vi "loadEntityTransaction.vi"() -> ()   [LabVIEW 2012]
uses:
  <vilib>/addons/database/Connection.llb/DB Tools Open Connec (Path).vi
  <vilib>/addons/database/Connection.llb/Conn Execute.vi
  <vilib>/addons/database/Recordset.llb/Rec Fetch Recordset Data (R).vi
  <vilib>/addons/database/Recordset.llb/Rec Destroy - Connection.vi
  <vilib>/addons/database/_DB Variant To Data/Database Variant To Data.xnode
  <vilib>/addons/database/NI_Database_API.lvlib
panel:
  out "recordset data":variant[][](array[variant])
  out "error out 3":errorcluster
  out "data 2":string
  out "error out 2":errorcluster
  in  "Cluster":T1
  out "concatenated string":string
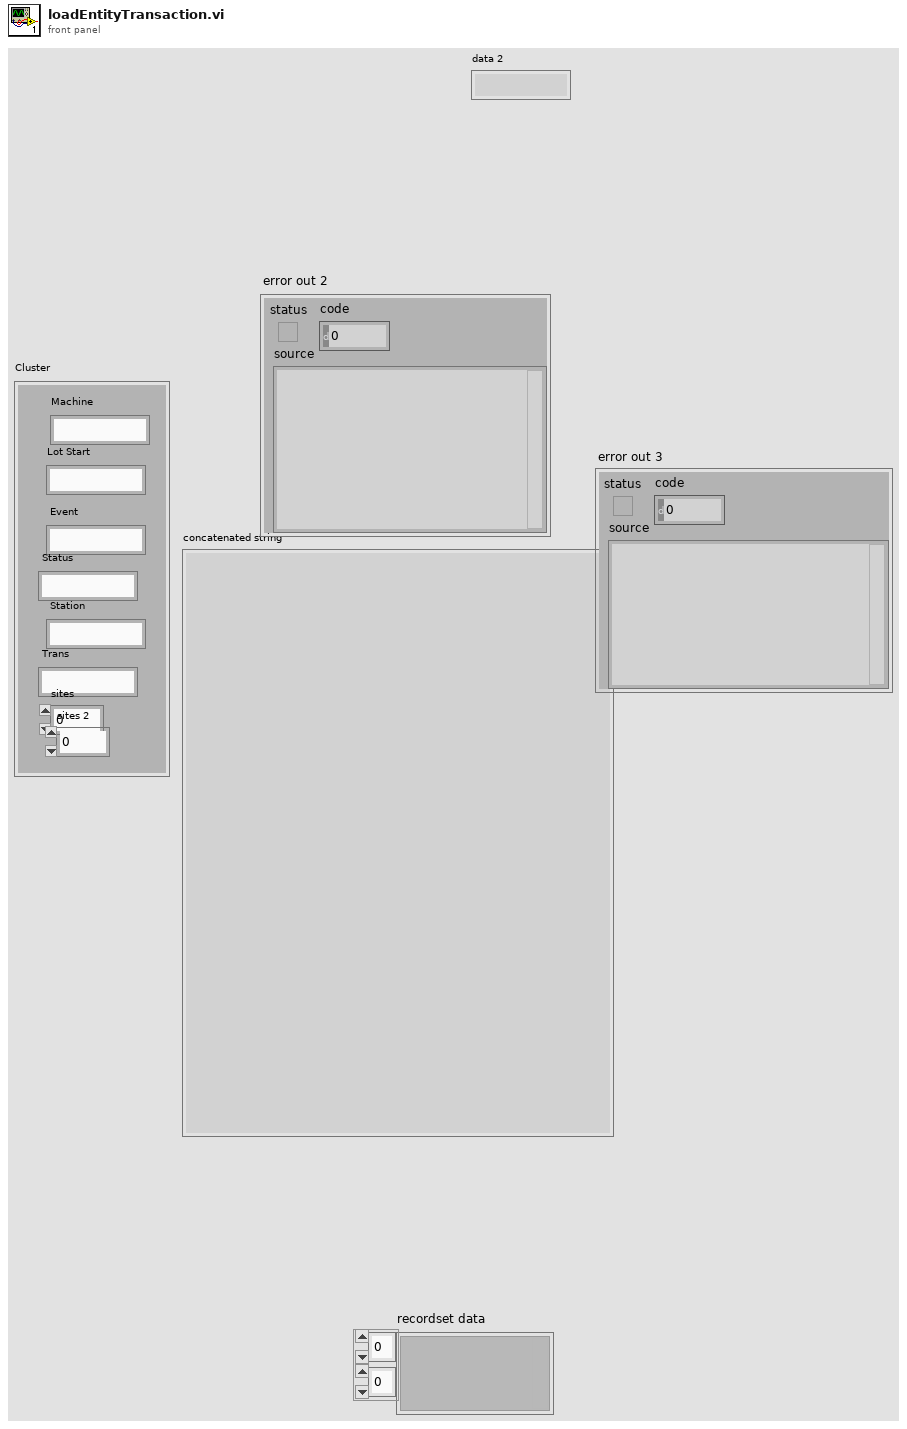
[diagram p1: front panel]
types:
  T1 = cluster{"Machine":string, "Lot Start":string, " Event":string, " Status":string, " Station":string, " Trans":string, "sites":dbl, "sites 2":dbl}
  T2 = typedef "NI_Database_API.lvlib/Conn ObjectReference.ctl" = refnum<k1>
  T3 = typedef "NI_Database_API.lvlib/Rec ObjectReference.ctl" = refnum<k1>
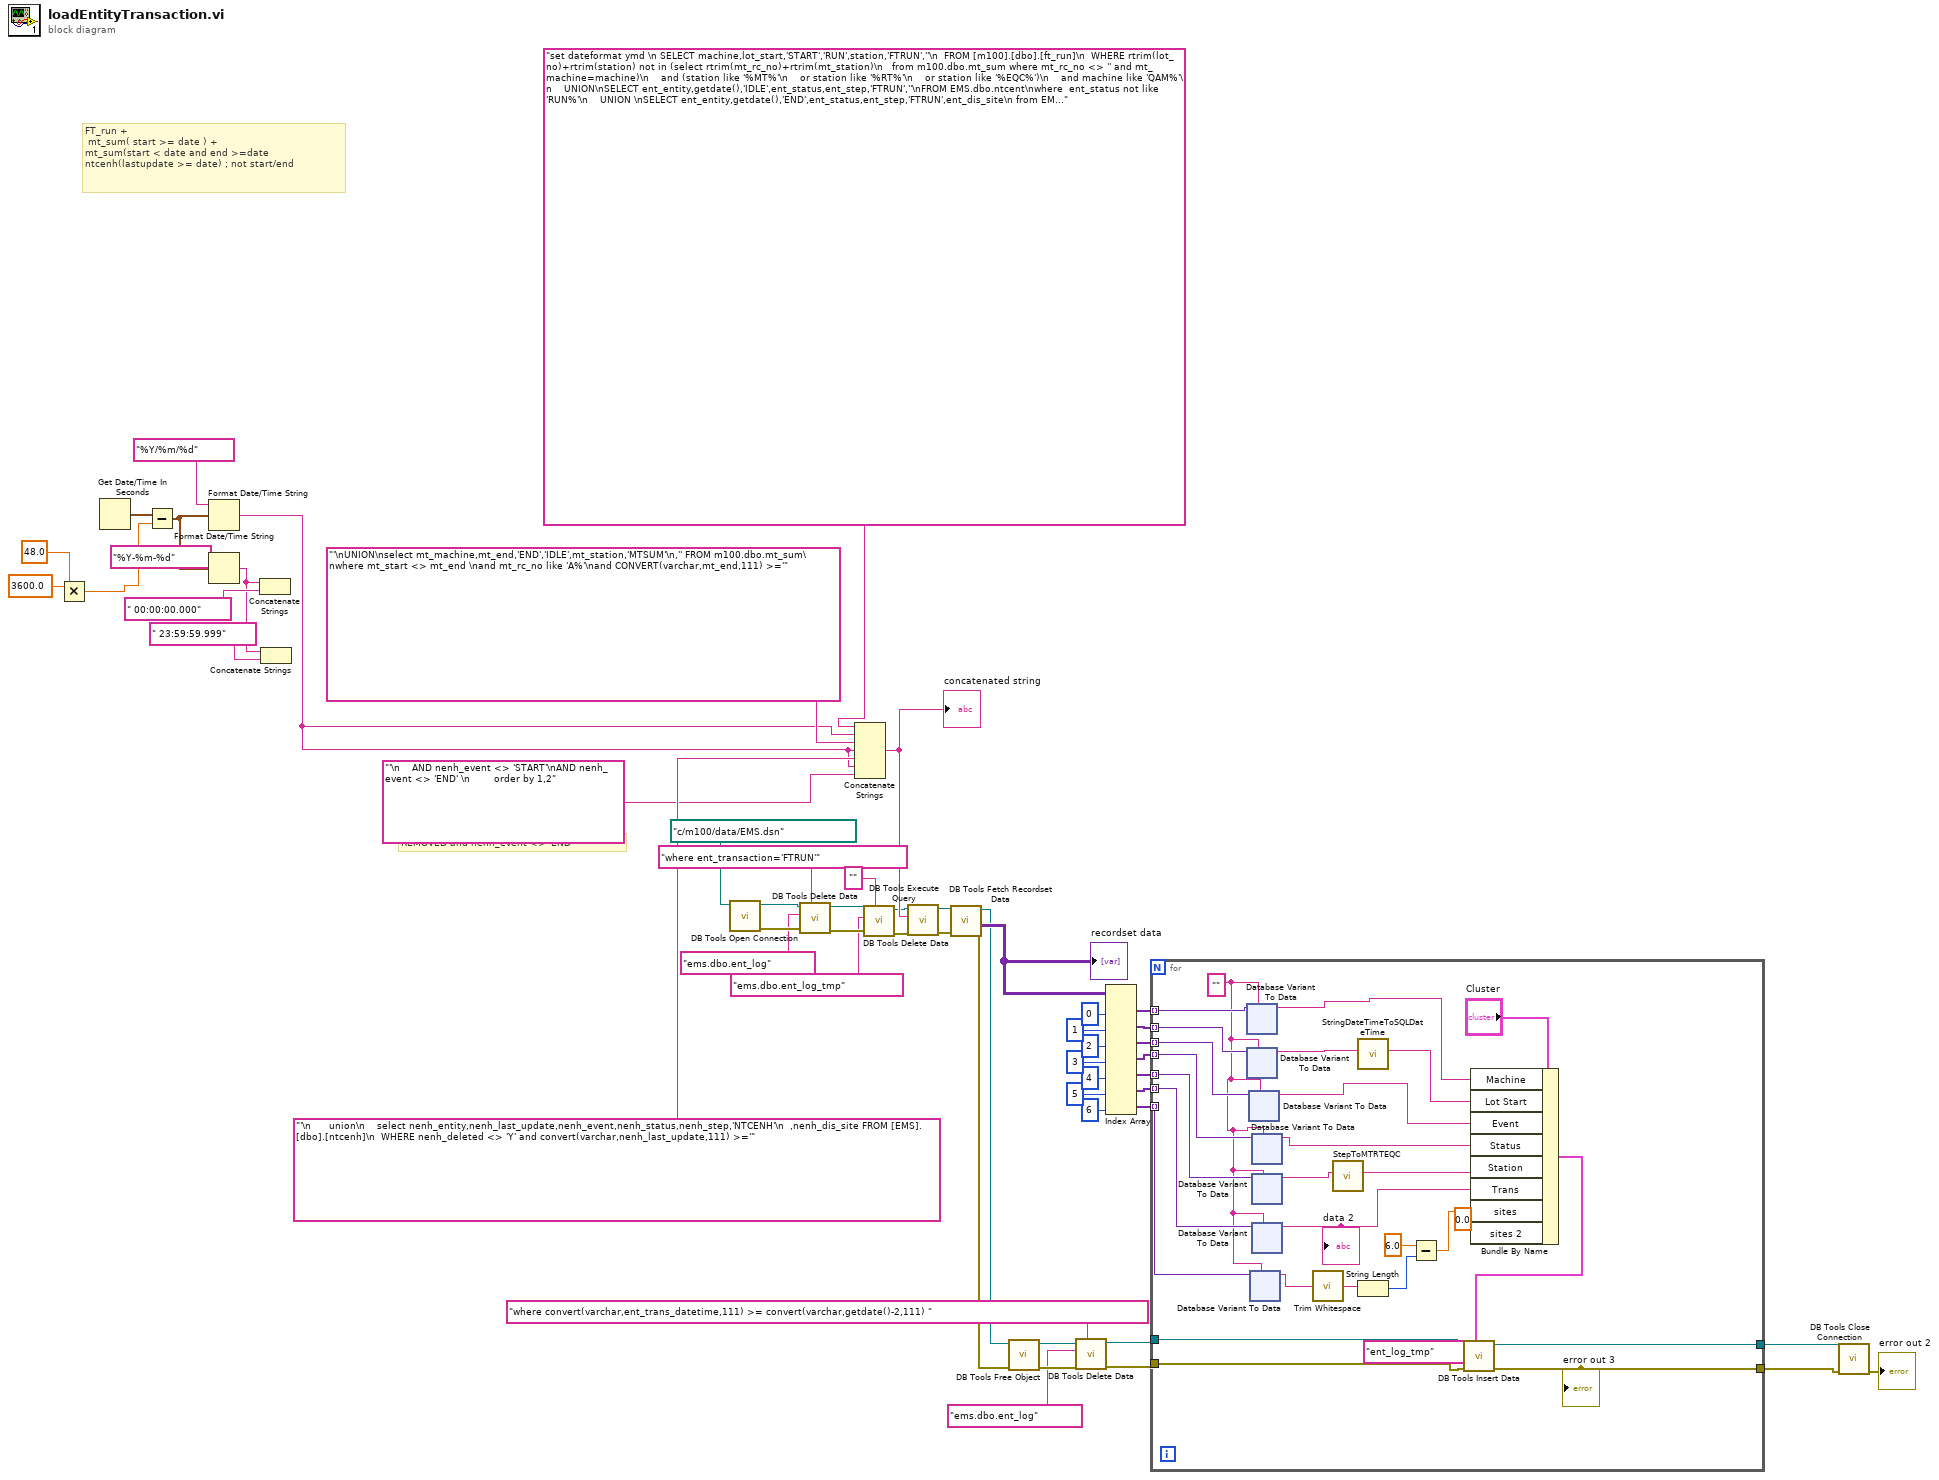
[diagram p0: block diagram]
diagram:
  # "REMOVED and nenh_event <> 'END'"
  # "FT_run +\n mt_sum( start >= date ) + \nmt_sum(start < date and end >=date\nntcenh(lastupdate >= date) ; not start/end"
  n1 = Multiply(x=3600.0, y=48.0) -> (x*y=w35:dbl)
  n2 = Get Date/Time In Seconds() -> (seconds since 1Jan1904=w38:timestamp)
  n3 = Subtract(x=w38, y=w35) -> (x-y=w33:timestamp)
  n4 = Format Date/Time String(time format string (%c)="%Y/%m/%d", seconds (now)=w33) -> (date/time string=w22:string)  [unwired: 1 in]
  n5 = Format Date/Time String(time format string (%c)="%Y-%m-%d", seconds (now)=w33) -> (date/time string=w30:string)  [unwired: 1 in]
  n6 = Concatenate Strings(w30, " 00:00:00.000" ("string")) -> ()  [unwired: 1 out]
  n7 = Concatenate Strings(w30, " 23:59:59.999" ("string")) -> ()  [unwired: 1 out]
  n8 = call-poly <vilib>:"DB Tools Open Connection.vi"("connection information"=path "c:/m100/data/EMS.dsn") -> ("error out"=w18:errorcluster, "connection reference"=w20:T2)  [unwired: 7 in]
  n9 = call <vilib>:"DB Tools Delete Data.vi"("condition"="where ent_transaction='FTRUN'", "error in (no error)"=w18, "table"="ems.dbo.ent_log", "connection reference"=w20) -> ("error out"=w17:errorcluster, "connection reference out"=w19:T2)  [unwired: 6 in]
  n10 = Concatenate Strings("set dateformat ymd \n SELECT machine,lot_start,'START','RUN',station,'FTRUN',''\n  FROM [m100].[dbo].[ft_run]\n  WHERE rtrim(lot_no)+rtrim(station) not in (select rtrim(mt_rc_no)+rtrim(mt_station)\n   from m100.dbo.mt_sum where mt_rc_no <> '' and mt_machine=machine)\n    and (station like '%MT%'\n    or station like '%RT%'\n    or station like '%EQC%')\n    and machine like 'QAM%'\n    UNION\nSELECT ent_entity,getdate(),'IDLE',ent_status,ent_step,'FTRUN',''\nFROM EMS.dbo.ntcent\nwhere  ent_status not like 'RUN%'\n    UNION \nSELECT ent_entity,getdate(),'END',ent_status,ent_step,'FTRUN',ent_dis_site\n from EMS.dbo.ntcent\nwhere ent_status like 'RUN%'\n    UNION\n    SELECT mt_machine,mt_start,'START','RUN',mt_station,'MTSUM'\n    ,'' FROM m100.dbo.mt_sum\n    where mt_start <> mt_end \nand mt_rc_no like 'A%'\nand CONVERT(varchar,mt_start,111) >='", w22, "'\nUNION\nselect mt_machine,mt_end,'END','IDLE',mt_station,'MTSUM'\n,'' FROM m100.dbo.mt_sum\nwhere mt_start <> mt_end \nand mt_rc_no like 'A%'\nand CONVERT(varchar,mt_end,111) >='" ("string"), w22, "'\n      union\n    select nenh_entity,nenh_last_update,nenh_event,nenh_status,nenh_step,'NTCENH'\n  ,nenh_dis_site FROM [EMS].[dbo].[ntcenh]\n  WHERE nenh_deleted <> 'Y' and convert(varchar,nenh_last_update,111) >='" ("string"), w22, "'\n    AND nenh_event <> 'START'\nAND nenh_event <> 'END' \n        order by 1,2" ("string")) -> (w52:string)
  "concatenated string" <- w52
  n11 = call <vilib>:"DB Tools Delete Data.vi"("condition"="", "error in (no error)"=w17, "table"="ems.dbo.ent_log_tmp", "connection reference"=w19) -> ("error out"=w16:errorcluster, "connection reference out"=w11:T2)  [unwired: 6 in]
  n12 = call-poly <vilib>:"DB Tools Execute Query.vi"("error in (no error)"=w16, "SQL query"=w52, "connection reference"=w11) -> ("error out"=w9:errorcluster, "recordset reference"=w10:T3)  [unwired: 5 in]
  n13 = call-poly <vilib>:"DB Tools Fetch Recordset Data.vi"("error in (no error)"=w9, "recordset reference"=w10) -> ("error out"=w7:errorcluster, "recordset data"=w51:variant[][], "recordset reference out"=w8:T3)  [unwired: 3 in]
  "recordset data" <- w51
  n14 = call-poly <vilib>:"DB Tools Free Object.vi"("error in (no error)"=w7, "recordset reference"=w8) -> ("error out"=w4:errorcluster, "connection reference"=w6:T2)  [unwired: 8 in]
  n15 = call <vilib>:"DB Tools Delete Data.vi"("condition"="where convert(varchar,ent_trans_datetime,111) >= convert(varchar,getdate()-2,111) ", "error in (no error)"=w4, "table"="ems.dbo.ent_log", "connection reference"=w6) -> ("error out"=w3:errorcluster, "connection reference out"=w5:T2)  [unwired: 6 in]
  n16 = Index Array(array=w51, index (col) #1=0 ("disabled index (col)"), index (col) #2=1 ("index (col)"), index (col) #3=2 ("index (col)"), index (col) #4=3 ("index (col)"), index (col) #5=4 ("index (col)"), index (col) #6=5 ("index (col)"), index (col) #7=6 ("index (col)")) -> (element #1=w44:variant[], element #2=w43:variant[], element #3=w42:variant[], element #4=w41:variant[], element #5=w40:variant[], element #6=w39:variant[], element #7=w24:variant[])  [unwired: 7 in]
  n17 = for {
    tunnel: w44 -> [w84] mode=indexing
    tunnel: w43 -> [w83] mode=indexing
    tunnel: w42 -> [w82] mode=indexing
    tunnel: w41 -> [w81] mode=indexing
    tunnel: w40 -> [w80] mode=indexing
    tunnel: w39 -> [w79] mode=indexing
    tunnel: w5 -> [w66]
    tunnel: [w73] -> w28
    tunnel: w3 -> [w72]
    tunnel: [w71] -> w27
    tunnel: w24 -> [w65] mode=indexing
    w64 = ""
    n18 = xnode "Database Variant To Data"("database variant"=w84, "type"=w64) -> ("data"=w77:string)  [unwired: 1 in, 1 out]
    n19 = xnode "Database Variant To Data"("database variant"=w83, "type"=w64) -> ("data"=w68:string)  [unwired: 1 in, 1 out]
    n20 = xnode "Database Variant To Data"("database variant"=w82, "type"=w64) -> ("data"=w76:string)  [unwired: 1 in, 1 out]
    n21 = xnode "Database Variant To Data"("database variant"=w65, "type"=w64) -> ("data"=w63:string)  [unwired: 1 in, 1 out]
    n22 = xnode "Database Variant To Data"("database variant"=w81, "type"=w64) -> ("data"=w75:string)  [unwired: 1 in, 1 out]
    n23 = xnode "Database Variant To Data"("database variant"=w80, "type"=w64) -> ("data"=w57:string)  [unwired: 1 in, 1 out]
    n24 = xnode "Database Variant To Data"("database variant"=w79, "type"=w64) -> ("data"=w74:string)  [unwired: 1 in, 1 out]
    "data 2" <- w74
    n25 = call <vilib>:"Trim Whitespace.vi"("string"=w63) -> ("trimmed string"=w62:string)  [unwired: 1 in]
    n26 = call "StepToMTRTEQC.vi"("StationIn"=w57) -> ("StationOut"=w56:string)  [unwired: 10 in]
    n27 = call "StringDateTimeToSQLDateTime.vi"("String"=w68) -> ("date/time string"=w67:string)  [unwired: 9 in, 1 out]
    n28 = String Length(string=w62) -> (length=w60:i32)
    n29 = Subtract(x=6.0, y=w60) -> (x-y=w59:dbl)
    n30 = Bundle By Name(cluster="Cluster", "Machine"=w77, "Lot Start"=w67, "Event"=w76, "Status"=w75, "Station"=w56, "Trans"=w74, "sites"=w59, "sites 2"=0.0) -> (w69:T1)
    n31 = call <vilib>:"DB Tools Insert Data.vi"("data"=w69, "error in (no error)"=w72, "table"="ent_log_tmp", "connection reference"=w66) -> ("error out"=w71:errorcluster, "connection reference out"=w73:T2)  [unwired: 6 in]
    "error out 3" <- w71
  }
  n32 = call <vilib>:"DB Tools Close Connection.vi"("error in (no error)"=w27, "connection reference"=w28) -> ("error out"=→"error out 2":errorcluster)  [unwired: 5 in]
